vi "Calculate Remote Sense Lead Resistance.vi"(8 "error in (no error)":errorcluster, 10 "Load Current (0 amperes)":dbl, 11 "VISA resource name":refnum<visa-resource-name>) -> (0 "error out":errorcluster, 3 "VISA resource name out":refnum<visa-resource-name>)   [LabVIEW 2018, in "XP Power PLS600.lvlib"]
doc: "Initiates calculation of the Remote Sense lead resistance at the specified load current. The current is specified in amperes."
uses:
  XP Power PLS600.lvlib
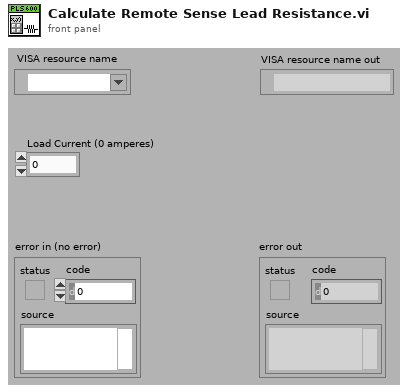
[diagram p1: front panel]
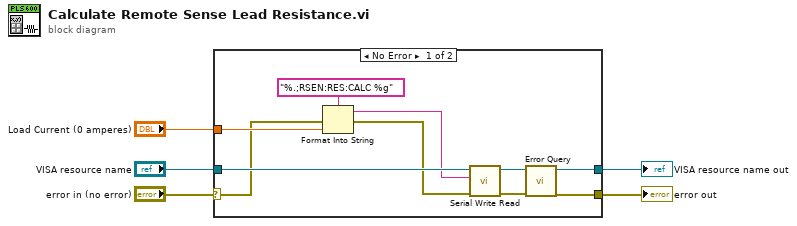
[diagram p0: block diagram]
diagram:
  n1 = case shown="No Error" "error in (no error)" {
    selector: "error in (no error)" -> [w7 w17]
    tunnel: [w15 w16] -> w5
    tunnel: [w14 w17] -> w4
    tunnel: "Load Current (0 amperes)" -> [w13 _]
    tunnel: "VISA resource name" -> [w12 w16]
    frame No Error {
      n2 = Format Into String(format string="%.;RSEN:RES:CALC %g", error in=w7, w13) -> (resulting string=w10:string, error out=w11:errorcluster)  [unwired: 1 in]
      n3 = call "Serial Write Read.vi"("error in (no error)"=w11, "Write Buffer"=w10, "VISA resource name"=w12) -> ("error out"=w8:errorcluster, "VISA resource name out"=w9:refnum<visa-resource-name>)  [unwired: 6 in, 1 out]
      n4 = call "Error Query.vi"("error in (no error)"=w8, "VISA resource name"=w9) -> ("error out"=w14:errorcluster, "VISA resource name out"=w15:refnum<visa-resource-name>)  [unwired: 6 in, 2 out]
    }
    frame Error {
    }
  }
  "VISA resource name out" <- w5
  "error out" <- w4
